vi "UDP config Sender.vi"(8 "error in (no error)":errorcluster, 11 "notifier out":refnum<notifier>) -> (0 "error out":errorcluster)   [LabVIEW 2014]
uses:
  PC_Functions.ctl
  <vilib>/Platform/TimedLoop/XDataNode/timing_clust.ctl
  <vilib>/Platform/TimedLoop/XDataNode/nitl_modes.ctl
  <vilib>/Platform/TimedLoop/XDataNode/wakeup.ctl
  <vilib>/Platform/TimedLoop/XDataNode/XDataNode.xnode
  <vilib>/Platform/TimedLoop/XDataNode/XDNodeRunTimeDep.lvlib
panel:
  out "connection error?":bool
  out "dt":u32
  in  "Cluster":T1={"local port"=5559, "receiver address"=0, "connection ID"=refnum, "receiver port"=5559}
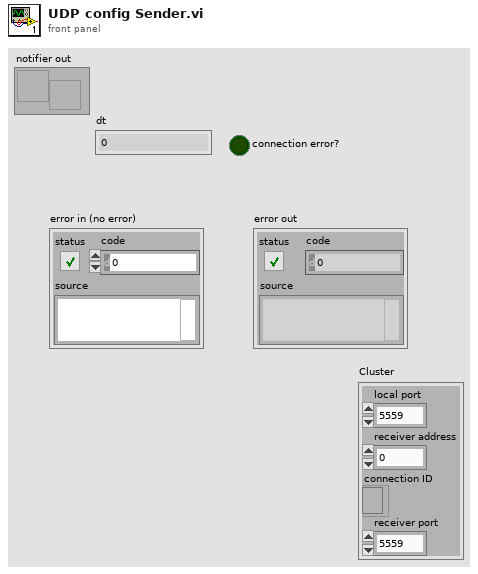
[diagram p1: front panel]
types:
  T1 = cluster{"local port":u16, "receiver address":u32, "connection ID":refnum<k16>, "receiver port":u16}
  T2 = typedef "PC_Functions.ctl" = enum16{"Initialize", "Send", "Idle", "Exit"}
  T3 = typedef "XDNodeRunTimeDep.lvlib/timing_clust.ctl" = cluster{"Expected End [f-1]":u64, "Actual End [f-1]":u64, "Finished Late? [f-1]":bool, "Expected End [i-1]":u64, "Actual End [i-1]":u64, "Finished Late? [i-1]":bool, "Expected Start [i]":u64, "Actual Start [i]":u64, "Expected Start [f]":u64, "Actual Start [f]":u64, "Source Name":string, "Structure Name":string, "Period":i64, "Deadline":i64, "Offset":i64, "Start":i64, "Priority":i32, "Timeout":i32, "Mode":T4, "Wakeup Reason":T5, "Error":errorcluster, "Source Type":string, "Secondary Source Type":string, "Global End Time":u64, "Global Start Time":u64, "Frame Duration":u64, "Iteration Duration":u64, "Assigned CPU":i32, "I/O Scan Engine Mode":u32}
  T4 = typedef "XDNodeRunTimeDep.lvlib/nitl_modes.ctl" = enum32{"No Change", "Process missed periods, maintain original phase", "Discard missed periods, maintain original phase", "Process missed periods, ignore original phase", "Discard missed periods, ignore original phase"}
  T5 = typedef "XDNodeRunTimeDep.lvlib/wakeup.ctl" = enum32{"Normal", "Aborted", "Asynchronous wakeup", "Timing source error", "Timed loop error", "Timeout"}
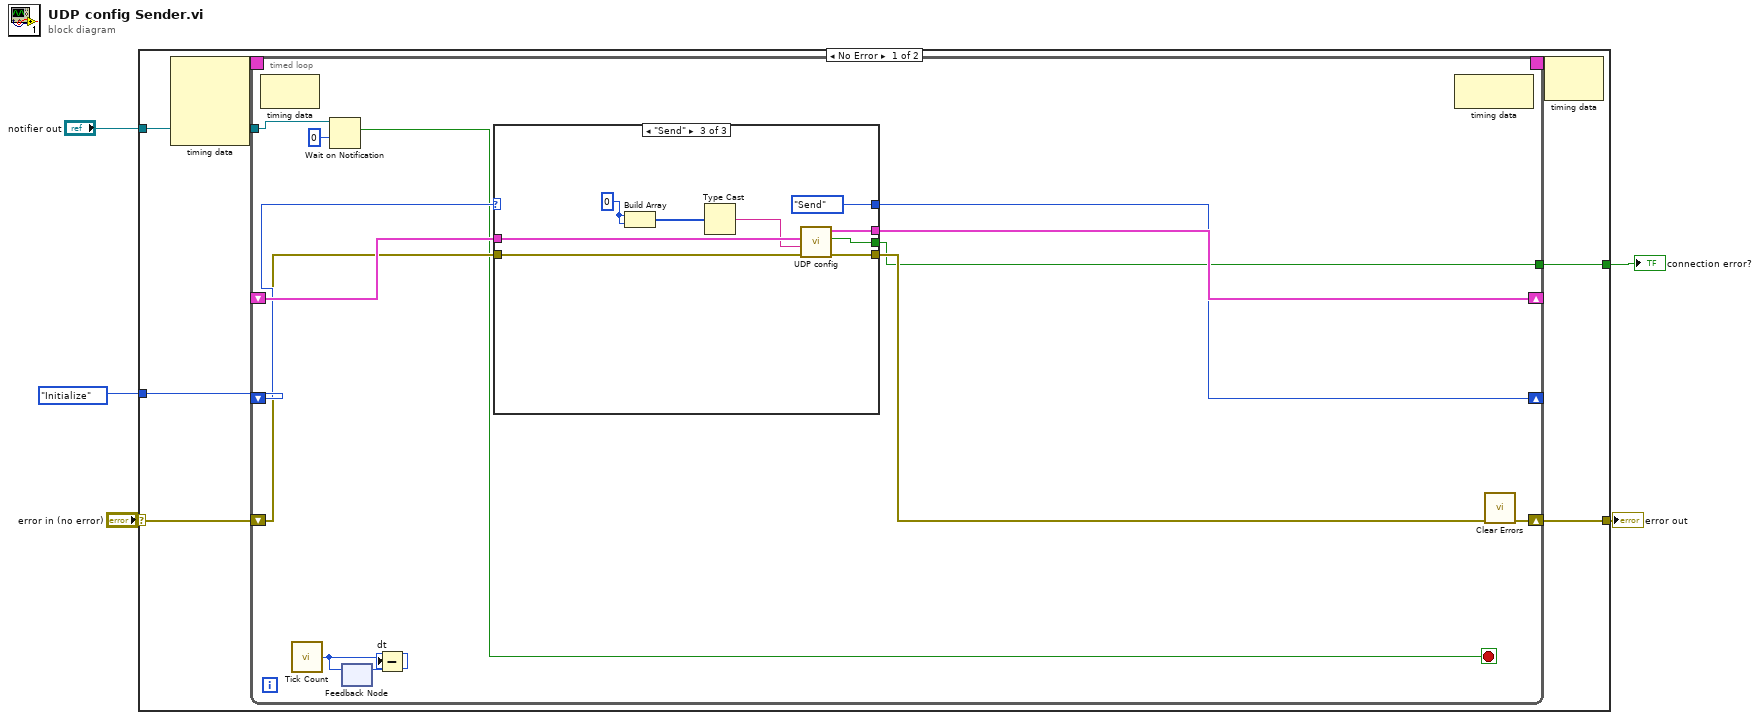
[diagram p0: block diagram]
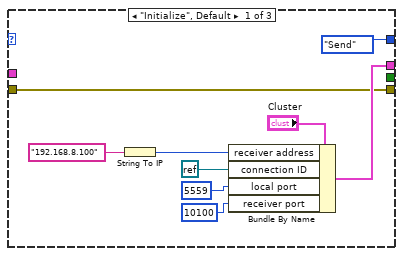
[diagram p2: hidden frame]
diagram:
  n1 = case shown="No Error" "error in (no error)" {
    selector: "error in (no error)" -> [w11 w52]
    tunnel: [w12 w52] -> w4
    tunnel: PC_Functions."Initialize" ("Command") -> [w10 _]
    tunnel: [w9 _] -> w3
    tunnel: "notifier out" -> [w8 _]
    frame No Error {
      n2 = node-c288() -> (w7:T3)  [unwired: 4 in]
      n3 = timed-loop {
        shift-right: [w24] -> w12
        shift-left: w11 -> [w16]
        shift-right: [w26] -> _
        shift-left: _ -> [w25]
        shift-right: [w19] -> _
        shift-left: w10 -> [w17]
        tunnel: [w18] -> w9
        tunnel: w8 -> [w14]
        timing: w7 -> [_]
        timing-out: [_] -> w6
        stop <- w13 stop-if-true
        n4 = node-c288() -> ()  [unwired: 1 in, 1 out]
        n5 = call "Tick Count"() -> ("Tick Count(uSec)"=w21:u32)
        n6 = Wait on Notification(notifier=w14, timeout in ms (-1)=0) -> (notification=w13:bool)  [unwired: 2 in, 3 out]
        n7 = feedback #1() -> (w22:u32)  [unwired: 1 in]
        n8 = feedback-in #1(w21) -> ()
        n9 = Subtract(x=w21, y=w22) -> (x-y=→"dt":u32)
        n10 = case shown="\"Send\"" w17 {
          selector: w17 -> [_ w39 _]
          tunnel: [w32 w40 w45] -> w26
          tunnel: w25 -> [_ w40 w48]
          tunnel: w16 -> [w31 w38 w42]
          tunnel: [w31 w38 w43] -> w23
          tunnel: [PC_Functions."Send" ("Command") w39 PC_Functions."Send" ("Command")] -> w19
          tunnel: [_ _ w46] -> w18
          frame "Initialize", Default {
            n11 = String To IP(1:"192.168.8.100" ("receiver address")) -> (0:w35:u32)
            n12 = Bundle By Name(cluster="Cluster", "receiver address"=w35, "connection ID"=refnum<k0> refnum, "local port"=u16 5559, "receiver port"=u16 10100) -> (w32:T1)
          }
          frame "Idle" {
          }
          frame "Send" {
            w44 = u32 0
            n13 = Build Array(w44, w44) -> (w41:u32[])
            n14 = Type Cast(x=w41) -> (*(type *) &x=w47:string)  [unwired: 1 in]
            n15 = call "UDP config.vi"("error in"=w42, "message"=w47, "Cluster in"=w48) -> ("error out"=w43:errorcluster, "connection error?"=w46:bool, "Cluster out"=w45:T1)  [unwired: 5 in, 1 out]
          }
        }
        n16 = node-c288() -> ()  [unwired: 1 in, 1 out]
        n17 = call <vilib>:"Clear Errors.vi"("error in (no error)"=w23) -> ("error out"=w24:errorcluster)  [unwired: 5 in, 1 out]
      }
      n18 = node-c288(w6) -> ()  [unwired: 1 out]
    }
    frame Error {
    }
  }
  "error out" <- w4
  "connection error?" <- w3
